vi "Update Array.vi"(8 "error in (no error)":errorcluster, 10 "Array":dbl[](array[numeric]), 11 "Example View In":refnum<class "Example View Actor.lvclass">) -> (0 "error out":errorcluster, 3 "Example View Out":refnum<class "Example View Actor.lvclass">)   [LabVIEW 2023, in "Example Event Actors.lvlib" / "Example View Actor.lvlib" / "Example View Actor.lvclass"]
uses:
  Example View Actor.lvclass
  Example View Actor.lvclass/Example View Actor.ctl
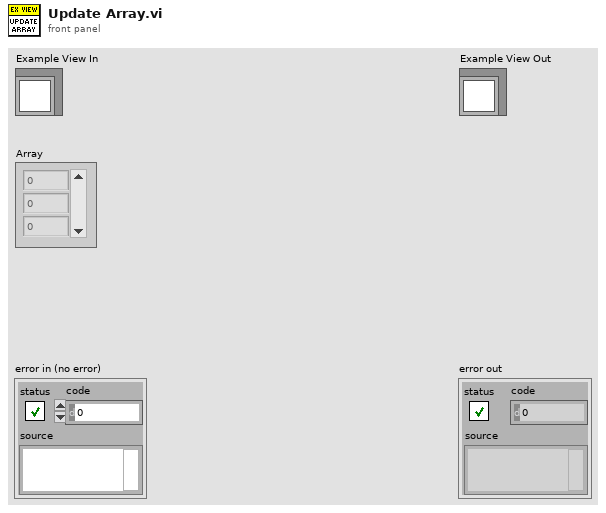
[diagram p1: front panel]
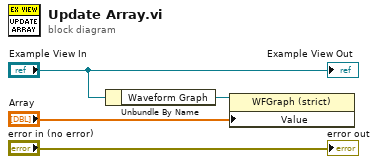
[diagram p0: block diagram]
diagram:
  n1 = Unbundle By Name("Example View In") -> ("Waveform Graph"=w2:refnum<vi>)
  n2 = property class="WFGraph (strict)"(reference=w2, "Value"="Array") -> ()  [unwired: 1 in, 2 out]
  "error out" <- "error in (no error)"
  "Example View Out" <- "Example View In"
